vi "Variant Constant (empty object).vi"() -> (1 "Empty Object":variant)   [LabVIEW 2015]
doc: "Void variant representing empty object (\"{}\"). \n\nUsed for representing JSON objects.\n\nTo read/write/removes key:value pairs to the object, use the variant attribute manipulation functions."
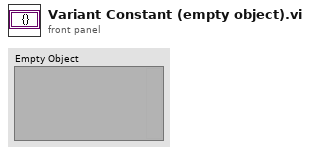
[diagram p1: front panel]
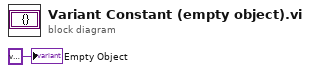
[diagram p0: block diagram]
diagram:
  "Empty Object" <- variant
